vi "DisconncetFromDatabase.vi"(8 "error in":errorcluster, 11 "Database ref":refnum<k24>) -> (0 "error out":errorcluster)   [LabVIEW 2015]
uses:
  C:/Users/Bartek/Desktop/NORDIC Labview GUI/DLLs/NordicDatabaseDLL.dll
  DLLs/NordicDatabaseDLL.dll
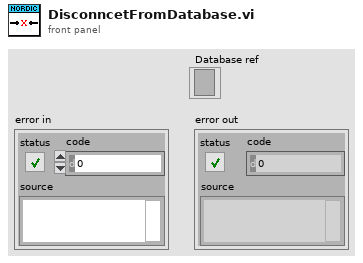
[diagram p1: front panel]
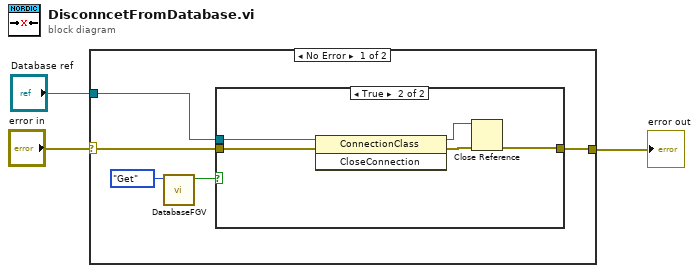
[diagram p0: block diagram]
diagram:
  n1 = case shown="No Error" "error in" {
    selector: "error in" -> [w8 w15]
    tunnel: [w7 w15] -> w2
    tunnel: "Database ref" -> [w4 _]
    frame No Error {
      n2 = call "DatabaseFGV.vi"("State"=enum16{"Get", "Set"}."Get") -> ("Active?"=w5:bool)  [unwired: 10 in]
      n3 = case shown="True" w5 {
        tunnel: w8 -> [w9 w12]
        tunnel: [w9 w11] -> w7
        tunnel: w4 -> [_ w10]
        frame False {
        }
        frame True {
          n4 = invoke class="ConnectionClass" method="CloseConnection"(reference=w10, error in=w12) -> (reference out=w13:refnum<k24>, error out=w14:errorcluster)  [unwired: 1 in, 1 out]
          n5 = Close Reference(reference=w13, error in (no error)=w14) -> (error out=w11:errorcluster)
        }
      }
    }
    frame Error {
    }
  }
  "error out" <- w2
